vi "BuildWorker Launcher.vi"(10 "Show":bool=TRUE, 11 "Port":u16=4545) -> (3 "Worker Enqueuer":refnum<class "Message Enqueuer.lvclass">)   [LabVIEW 2017]
uses:
  <vilib>/ActorFramework/Message Enqueuer/Message Enqueuer.lvclass
  <vilib>/ActorFramework/Message Enqueuer/Message Enqueuer.lvclass/Message Enqueuer.ctl
  <vilib>/ActorFramework/Message Enqueuer/Enqueue.vi
  Actors/BuildWorker/BuildWorker/BuildWorker.lvclass
  C:/Program Files (x86)/National Instruments/LabVIEW 2017/vi.lib/ActorFramework/Actor/Actor.lvclass
  Actors/Framework/Actor wUI Messages/Show UI Msg/Show UI Msg.lvclass
  C:/Program Files (x86)/National Instruments/LabVIEW 2017/vi.lib/ActorFramework/Message/Message.lvclass
  <vilib>/ActorFramework/Message Priority Queue/Priority Enqueue.vi
  <vilib>/ActorFramework/Actor/Actor.lvclass
panel:
  # "BuildWorker Launcher"
  # "\"C:\\Program Files (x86)\\National Instruments\\LabVIEW 2017\\LabVIEW.exe\" \"..\\BuildWorker Launcher.vi\" -- /diskLetter:A /buildServerPort:4545 /showWindow:FALSE"
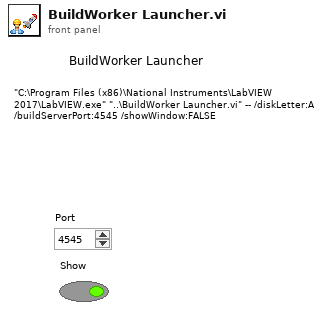
[diagram p1: front panel]
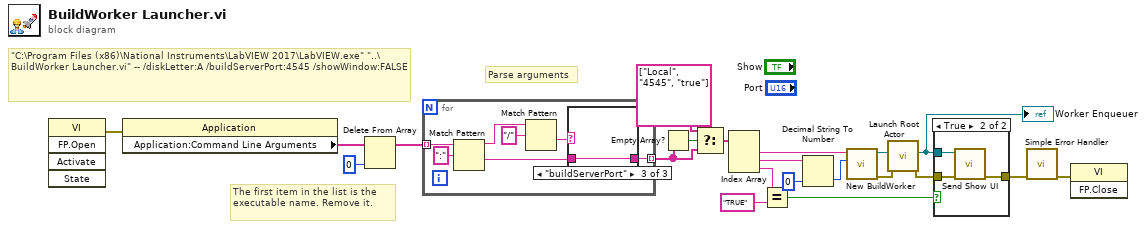
[diagram p0: block diagram]
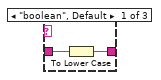
[diagram p3: hidden frame]
diagram:
  # "Parse arguments"
  # "\"C:\\Program Files (x86)\\National Instruments\\LabVIEW 2017\\LabVIEW.exe\" \"..\\BuildWorker Launcher.vi\" -- /diskLetter:A /buildServerPort:4545 /showWindow:FALSE"
  # "The first item in the list is the executable name. Remove it."
  n1 = invoke class="VI" method="FP.Open"() -> (error out=w5:errorcluster)  [unwired: 5 in, 4 out]
  n2 = property class="Application"(error in=w5) -> ("Application:Command Line Arguments"=w21:string[])  [unwired: 1 in, 2 out]
  n3 = Delete From Array(array=w21, index=0 ("length")) -> (array with subset deleted=w17:string[])  [unwired: 1 in, 1 out]
  n4 = for {
    tunnel: w17 -> [w27] mode=indexing
    tunnel: [w22] -> w8 mode=indexing
    n5 = Match Pattern(string=w27, regular expression=":") -> (before substring=w25:string, after substring=w26:string)  [unwired: 3 out]
    n6 = Match Pattern(string=w25, regular expression="/") -> (after substring=w23:string)  [unwired: 4 out]
    n7 = case shown="\"buildServerPort\"" w23 {
      tunnel: w26 -> [w30 w31 w32]
      tunnel: [w29 w31 w32] -> w22
      frame "boolean", Default {
        n8 = To Lower Case(string=w30) -> (all lower case string=w29:string)
      }
      frame "diskLetter" {
      }
      frame "buildServerPort" {
      }
    }
  }
  n9 = Empty Array?(array=w8) -> (empty?=w9:bool)
  n10 = Select(t=string[] ["Local", "4545", "true"], s=w9, f=w8) -> (s? t:f=w6:string[])
  n11 = Index Array(array=w6) -> (element #1=w12:string, element #2=w11:string, element #3=w16:string)  [unwired: 3 in]
  n12 = Equal?(x=w16, y="TRUE") -> (x = y?=w1:bool)
  n13 = Decimal String To Number(string=w11, default (0L)=u16 0 ("default (0 I32)")) -> (number=w2:u16)  [unwired: 1 in, 1 out]
  n14 = call "New BuildWorker.vi"("BuildServer Port"=w2, "Name"=w12) -> ("error out"=w18:errorcluster, "BuildWorker out"=w19:refnum<class "BuildWorker.lvclass">)  [unwired: 8 in]
  n15 = call <vilib>:"Launch Root Actor.vi"("error in (no error)"=w18, "Actor"=w19) -> ("error out"=w13:errorcluster, "Actor's Enqueuer"=w14:refnum<class "Message Enqueuer.lvclass">)  [unwired: 8 in]
  "Worker Enqueuer" <- w14
  n16 = case shown="True" w1 {
    tunnel: w14 -> [_ w36]
    tunnel: w13 -> [w33 w35]
    tunnel: [w33 w34] -> w4
    frame False {
    }
    frame True {
      n17 = call "Send Show UI.vi"("error in (no error)"=w35, "Message Enqueuer in"=w36) -> ("error out"=w34:errorcluster)  [unwired: 8 in, 1 out]
    }
  }
  n18 = call <vilib>:"Simple Error Handler.vi"("error in (no error)"=w4) -> ("error out"=w3:errorcluster)  [unwired: 4 in, 4 out]
  n19 = invoke class="VI" method="FP.Close"(error in=w3) -> ()  [unwired: 2 in, 3 out]
